vi "Is Path Valid and Exists.vi"(6 "Check Inside LLBs?":bool, 8 "File/Folder Path":path) -> (0 "Valid and Exists?":bool, 1 "Is Directory":bool)   [LabVIEW 2011]
doc: "This VI will return if a file or a folder exists and is a valid path. The <b>File/Folder Path</b> is used as the input and if the path is a directory <b>Is Directory?</b> will be set to TRUE. If the path provided is a valid path, and it the path exists, then the <b>Valid and Exists?</b> boolean will be set to TRUE.\n\nThis VI by default will not look inside LLB files to find a valid path. If <b>Check Inside LLBs?</b> is TRUE it will."
uses:
  <userlib>/_OpenG.lib/file/file.llb/File Exists - Scalar__ogtk.vi
  <userlib>/_OpenG.lib/file/file.llb/Valid Path - Traditional__ogtk.vi
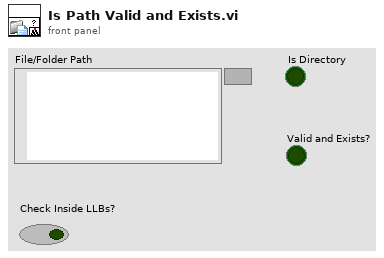
[diagram p1: front panel]
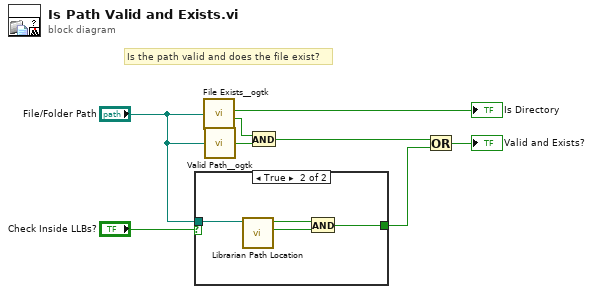
[diagram p0: block diagram]
diagram:
  # "Is the path valid and does the file exist?"
  n1 = case shown="True" "Check Inside LLBs?" {
    tunnel: "File/Folder Path" -> [_ w12]
    tunnel: [_ w9] -> w1
    frame False {
    }
    frame True {
      n2 = call <vilib>:"Librarian Path Location.vi"("path"=w12) -> ("path is to a file"=w10:bool, "path is in a VI library"=w11:bool)  [unwired: 6 in, 3 out]
      n3 = And(x=w11, y=w10) -> (x .and. y?=w9:bool)
    }
  }
  n4 = call-poly <userlib>:"File Exists__ogtk.vi"("file path"="File/Folder Path") -> ("is directory"=→"Is Directory":bool, "exists"=w7:bool)  [unwired: 6 in]
  n5 = call-poly <userlib>:"Valid Path__ogtk.vi"("path"="File/Folder Path") -> ("valid"=w8:bool)
  n6 = And(x=w7, y=w8) -> (x .and. y?=w5:bool)
  n7 = Or(x=w5, y=w1) -> (x .or. y?=→"Valid and Exists?":bool)
